vi "PPL_TRAJECTORY_EXECUTE_ABS.vi"(8 "Init":bool, 10 "Max Wheel Speed M/S":dbl, 11 "End Pose ENG":T6={"TRANSLATION"={"X"=0.0, "Y"=0.0}, "ROTATION"={"VALUE"=0.0, "COS"=1.0, "SIN"=0.0}} {"ROTATION"."SIN" format="%13.4f"; "ROTATION"."COS" format="%13.4f"; "ROTATION"."VALUE" format="%13.4f"; "TRANSLATION"."Y" format="%14.3f"; "TRANSLATION"."X" format="%14.3f"}) -> (0 "AtReference":bool, 2 "Right Speed Dmd M/S":dbl, 3 "Left Speed Dmd M/S":dbl)   [LabVIEW 2019]
uses:
  <vilib>/Rock Robotics/WPI/ThirdParty/JAS_Junk/TrajLib/TypeDef/POSE2D.ctl
  <vilib>/Rock Robotics/WPI/ThirdParty/JAS_Junk/TrajLib/TypeDef/TRANSLATION2D.ctl
  <vilib>/Rock Robotics/WPI/ThirdParty/JAS_Junk/TrajLib/TypeDef/ROTATION2D.ctl
  <vilib>/Rock Robotics/WPI/ThirdParty/MJansen/PathPlanner/TypeDef/PathPlannerTrajectory.ctl
  <vilib>/Rock Robotics/WPI/ThirdParty/MJansen/PathPlanner/TypeDef/PathPlannerTrajectoryState.ctl
  <vilib>/Rock Robotics/WPI/ThirdParty/MJansen/PathPlanner/TypeDef/PathPlannerPathConstraints.ctl
  <vilib>/Rock Robotics/WPI/ThirdParty/JAS_Junk/TrajLib/VI/Util_GetTime_U32.vi
  <vilib>/Rock Robotics/WPI/ThirdParty/JAS_Junk/TrajLib/Conv_Deg_Radians.vi
  <vilib>/Rock Robotics/WPI/ThirdParty/JAS_Junk/TrajLib/Rotation2d_GetRadians.vi
  <vilib>/Rock Robotics/WPI/ThirdParty/JAS_Junk/TrajLib/VI/Util_GetTime_U64.vi
  PPL_TRAJECTORY_GLOBALS.vi
  Diff_Drive_System/PPL_DRIVE_GLOBALS.vi
  <vilib>/Rock Robotics/WPI/ThirdParty/JAS_Junk/TrajLib/Trajectory_Library.lvlib
  <vilib>/Rock Robotics/WPI/ThirdParty/MJansen/PathPlanner/PathPlanner24.lvlib
panel:
  out "PathPlannerTrajectory":T1 {"States"."TargetHolonomicRotation"."SIN" format="%13.4f"; "States"."TargetHolonomicRotation"."COS" format="%13.4f"; "States"."TargetHolonomicRotation"."VALUE" format="%13.4f"; "States"."Heading"."SIN" format="%13.4f"; "States"."Heading"."COS" format="%13.4f"; "States"."Heading"."VALUE" format="%13.4f"; "States"."PositionMeters"."Y" format="%14.3f"; "States"."PositionMeters"."X" format="%14.3f"}
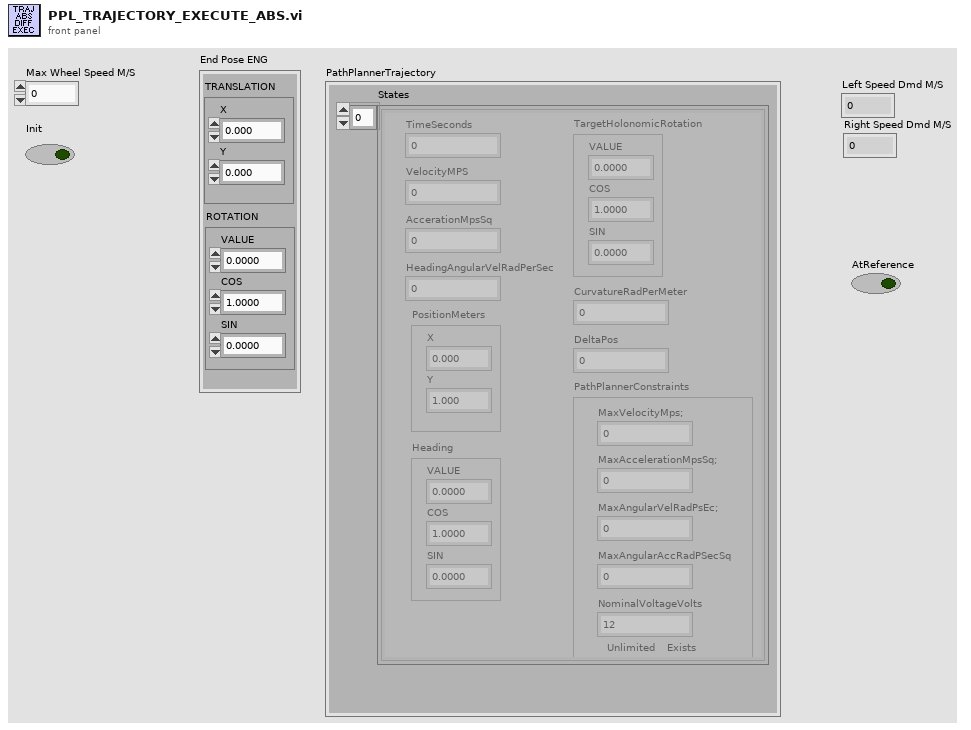
[diagram p1: front panel]
types:
  T1 = typedef "PathPlanner24.lvlib/PathPlannerTrajectory.ctl" = cluster{"States":T2[]}
  T2 = typedef "PathPlanner24.lvlib/PathPlannerTrajectoryState.ctl" = cluster{"TimeSeconds":dbl, "VelocityMPS":dbl, "AccerationMpsSq":dbl, "HeadingAngularVelRadPerSec":dbl, "PositionMeters":T3, "Heading":T4, "TargetHolonomicRotation":T4, "CurvatureRadPerMeter":dbl, "PathPlannerConstraints":T5, "DeltaPos":dbl}
  T3 = typedef "Trajectory_Library.lvlib/TRANSLATION2D.ctl" = cluster{"X":dbl, "Y":dbl}
  T4 = typedef "Trajectory_Library.lvlib/ROTATION2D.ctl" = cluster{"VALUE":dbl, "COS":dbl, "SIN":dbl}
  T5 = typedef "PathPlanner24.lvlib/PathPlannerPathConstraints.ctl" = cluster{"MaxVelocityMps;":dbl, "MaxAccelerationMpsSq;":dbl, "MaxAngularVelRadPsEc;":dbl, "MaxAngularAccRadPSecSq":dbl, "Exists":bool, "Unlimited":bool, "NominalVoltageVolts":dbl}
  T6 = typedef "Trajectory_Library.lvlib/POSE2D.ctl" = cluster{"TRANSLATION":T3, "ROTATION":T4}
  T7 = typedef "Trajectory_Library.lvlib/DIFF_DRIVE_KINEMATICS.ctl" = cluster{"TrackWidth_Meters":dbl}
  T8 = typedef "Trajectory_Library.lvlib/LTV_UNICYCLE_CONTROLLER_MODEL_PARAMS.CTL" = cluster{"Max linear ctrl effort M/S":dbl, "Max angular ctrl effort Rad/S":dbl, "Max Heading Meas Tol Rad":dbl, "Max X Pos Meas Tol M":dbl, "Max Y Pos Meas Tol M":dbl, "Max Linear Vel M/S":dbl}
  T9 = typedef "PathPlanner24.lvlib/PathPlannerCtrlLTVUnicycleConfig.ctl" = cluster{"Max Wheel Speed M/S":dbl, "Track Width M":dbl, "LTV_Unicycle_Ctrl_Model":T8, "LTV_Unicycle_Ctrl_Tolerance":T10}
  T10 = typedef "Trajectory_Library.lvlib/LTV_UNICYCLE_CONTROLLER_TOLERANCE.CTL" = cluster{"Max Heading Tolerance Rad":dbl, "Max X Tolerance M":dbl, "Max Y Tolerance M":dbl}
  T11 = typedef "Trajectory_Library.lvlib/LTV_UNICYCLE_CONTROLLER.ctl" = cluster{"States":i32, "Inputs":i32, "PoseError":T6, "PoseTolerance":T6, "Dt":dbl, "Enabled":bool, "LQR_K_Table":T12}
  T12 = typedef "Trajectory_Library.lvlib/FUNCTION_GENERATOR_MATRIX.ctl" = cluster{"Table Xs":dbl[], "Table Ys":variant[], "MinX":dbl, "MaxX":dbl, "ItemCount":i32, "Rows":i32, "Columns":i32}
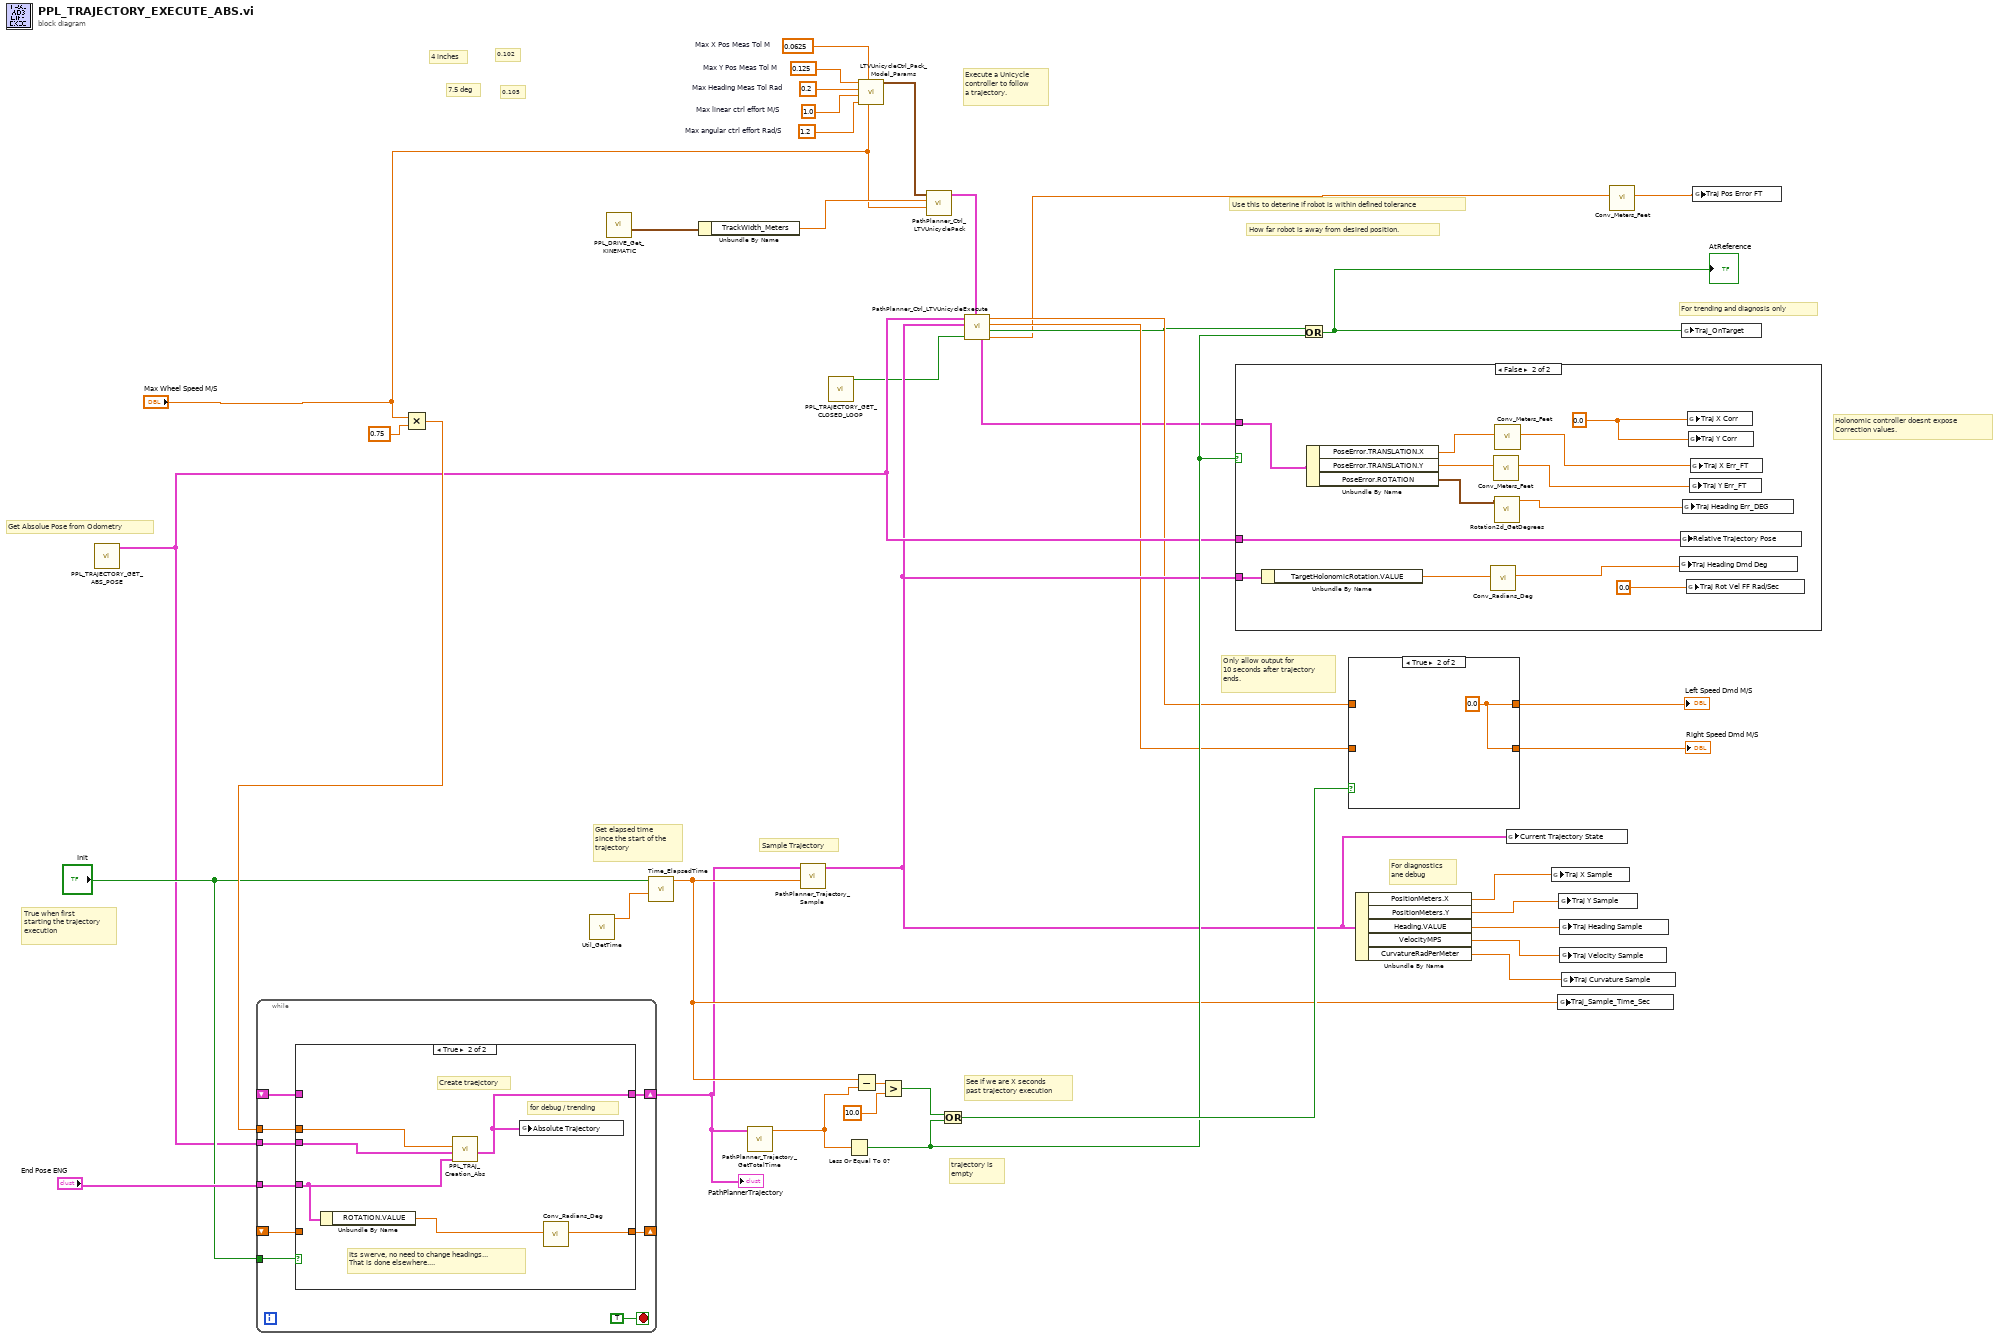
[diagram p0: block diagram]
diagram:
  w15 = 0.125  # Max Y Pos Meas Tol M
  w14 = 0.2  # Max Heading Meas Tol Rad
  w13 = 1.0  # Max linear ctrl effort M/S
  w12 = 1.2  # Max angular ctrl effort Rad/S
  w11 = 0.0625  # Max X Pos Meas Tol M
  # "0.105"
  # "0.102"
  # "Execute a Unicycle\ncontroller to follow\na trajectory."
  # "How far robot is away from desired position."
  # "Use this to deterine if robot is within defined tolerance"
  # "4 inches"
  # "7.5 deg"
  # "trajectory is \nempty"
  # "True when first\nstarting the trajectory\nexecution"
  # "Get elapsed time\nsince the start of the\ntrajectory"
  # "Holonomic controller doesnt expose\nCorrection values."
  # "For trending and diagnosis only"
  # "For diagnostics\nane debug"
  # "Get Absolue Pose from Odometry"
  # "Sample Trajectory"
  # "See if we are X seconds \npast trajectory execution"
  # "Only allow output for\n10 seconds after trajectory\nends."
  n1 = call "PPL_TRAJECTORY_GET_ABS_POSE.vi"() -> ("Absolute Odometry Pose"=w10:T6)  [unwired: 11 in]
  n2 = Multiply(x="Max Wheel Speed M/S", y=0.75) -> (x*y=w24:dbl)
  n3 = while {
    tunnel: "Init" -> [w48]
    tunnel: w10 -> [w47]
    shift-right: [w46] -> w26
    shift-left: _ -> [w45]
    shift-right: [w44] -> _
    shift-left: _ -> [w43]
    tunnel: "End Pose ENG" -> [w42]
    tunnel: w24 -> [w41]
    stop <- TRUE stop-if-true
    n4 = case shown="True" w48 {
      tunnel: w47 -> [_ w53]
      tunnel: [w51 w54] -> w46
      tunnel: w45 -> [w51 _]
      tunnel: [w50 w56] -> w44
      tunnel: w43 -> [w50 _]
      tunnel: w42 -> [_ w57]
      tunnel: w41 -> [_ w52]
      frame False {
      }
      frame True {
        # "for debug / trending"
        # "Its swerve, no need to change headings...\nThat is done elsewhere...."
        # "Create traejctory"
        n5 = Unbundle By Name(w57) -> ("ROTATION.VALUE"=w55:dbl)
        n6 = call "PPL_TRAJ_Creation_Abs.vi"("End Pose  ENG"=w57, "Current Pose SI"=w53, "Max Velocity M/S"=w52) -> ("PathPlannerTrajectory"=w54:T1)  [unwired: 6 in, 2 out]
        n7 = global write "PPL_TRAJECTORY_GLOBALS.vi" "Absolute Trajectory"(w54) -> ()
        n8 = call <vilib>:"Conv_Radians_Deg.vi"("Radians"=w55) -> ("Degrees"=w56:dbl)  [unwired: 10 in]
      }
    }
  }
  "PathPlannerTrajectory" <- w26
  n9 = call <vilib>:"Util_GetTime.vi"() -> ("FPGA_Time_Seconds"=w38:dbl)  [unwired: 9 in, 2 out]
  n10 = call "PPL_DRIVE_Get_KINEMATIC.vi"() -> ("out DIFF_DRIVE_KINEMATICS"=w21:T7)  [unwired: 11 in]
  n11 = call <vilib>:"Time_ElapsedTime.vi"("PassthroughTime_SEC"=w38, "Reset"="Init") -> ("Elapsed Time Sec"=w27:dbl)  [unwired: 9 in]
  n12 = Unbundle By Name(w21) -> ("TrackWidth_Meters"=w8:dbl)
  n13 = call <vilib>:"PathPlanner_Trajectory_GetTotalTime.vi"("PathPlannerTrajectory"=w26) -> ("TotalTimeSeconds"=w25:dbl)  [unwired: 10 in]
  n14 = call <vilib>:"PathPlanner_Trajectory_Sample.vi"("Time"=w27, "PathPlannerTrajectory"=w26) -> ("PathPlannerState"=w9:T2)  [unwired: 9 in]
  n15 = call "PPL_TRAJECTORY_GET_CLOSED_LOOP.vi"() -> ("AUTO_CLOSED_LOOP"=w7:bool)  [unwired: 11 in]
  n16 = Less Or Equal To 0?(x=w25) -> (x <= 0?=w28:bool)
  n17 = Subtract(x=w27, y=w25) -> (x-y=w40:dbl)
  n18 = call <vilib>:"LTVUnicycleCtrl_Pack_Model_Params.vi"("Max Linear Vel M/S"="Max Wheel Speed M/S", "Max X Pos Meas Tol M"=w11, "Max angular ctrl effort Rad/S"=w12, "Max linear ctrl effort M/S"=w13, "Max Heading Meas Tol Rad"=w14, "Max Y Pos Meas Tol M"=w15) -> ("LTV_Unicycle_Ctrl_Model _Params"=w17:T8)  [unwired: 5 in]
  n19 = Greater?(x=w40, y=10.0) -> (0:w31:bool)
  n20 = call <vilib>:"PathPlanner_Ctrl_LTVUnicyclePack.vi"("Max Speed M/S"="Max Wheel Speed M/S", "Track Width Meters"=w8, "LTV_Unicycle_Ctrl_Model"=w17) -> ("PathPlanner_Ctrl_LTVUnicycleConfig"=w16:T9)  [unwired: 8 in]
  n21 = Or(x=w31, y=w28) -> (x .or. y?=w30:bool)
  n22 = call <vilib>:"PathPlanner_Ctrl_LTVUnicycleExecute.vi"("PathPlanner_Ctrl_LTVUnicycle_Config"=w16, "Enabled"=w7, "PathPlannerState"=w9, "Current Pose SI"=w10) -> ("Position Error M"=w2:dbl, "At Reference"=w3:bool, "Normalized Right Wheel Dmd M/S"=w4:dbl, "Normalized Left Wheel Dmd M/S"=w5:dbl, "out LTV_UNICYCLE_CONTROLLER"=w1:T11)  [unwired: 3 in]
  n23 = case shown="False" w28 {
    tunnel: w10 -> [_ w61]
    tunnel: w9 -> [_ w64]
    tunnel: w1 -> [_ w58]
    frame True {
    }
    frame False {
      w70 = 0.0 ("Y Corr")
      n24 = Unbundle By Name(w64) -> ("TargetHolonomicRotation.VALUE"=w63:dbl)
      n25 = Unbundle By Name(w58) -> ("PoseError.TRANSLATION.X"=w66:dbl, "PoseError.TRANSLATION.Y"=w65:dbl, "PoseError.ROTATION"=w59:T4)
      n26 = call <vilib>:"Conv_Radians_Deg.vi"("Radians"=w63) -> ("Degrees"=w62:dbl)  [unwired: 10 in]
      n27 = call <vilib>:"Conv_Meters_Feet.vi"("Meters"=w65) -> ("Feet"=w69:dbl)  [unwired: 10 in]
      n28 = call <vilib>:"Rotation2d_GetDegrees.vi"("in ROTATION"=w59) -> ("AngleDegrees"=w60:dbl)  [unwired: 10 in]
      n29 = call <vilib>:"Conv_Meters_Feet.vi"("Meters"=w66) -> ("Feet"=w68:dbl)  [unwired: 10 in]
      n30 = global write "PPL_TRAJECTORY_GLOBALS.vi" "Traj Heading Dmd Deg"(w62) -> ()
      n31 = global write "PPL_TRAJECTORY_GLOBALS.vi" "Relative Trajectory Pose"(w61) -> ()
      n32 = global write "PPL_TRAJECTORY_GLOBALS.vi" "Traj Heading Err_DEG"(w60) -> ()
      n33 = global write "PPL_TRAJECTORY_GLOBALS.vi" "Traj Rot Vel FF Rad/Sec"(0.0 ("Traj Heading Dmd Deg")) -> ()
      n34 = global write "PPL_TRAJECTORY_GLOBALS.vi" "Traj X Corr"(w70) -> ()
      n35 = global write "PPL_TRAJECTORY_GLOBALS.vi" "Traj Y Corr"(w70) -> ()
      n36 = global write "PPL_TRAJECTORY_GLOBALS.vi" "Traj Y Err_FT"(w69) -> ()
      n37 = global write "PPL_TRAJECTORY_GLOBALS.vi" "Traj X Err_FT"(w68) -> ()
    }
  }
  n38 = Or(x=w3, y=w28) -> (x .or. y?=w29:bool)
  "AtReference" <- w29
  n39 = case shown="True" w30 {
    tunnel: w5 -> [w72 _]
    tunnel: [w72 w73] -> w20
    tunnel: w4 -> [w71 _]
    tunnel: [w71 w73] -> w19
    frame False {
    }
    frame True {
      w73 = 0.0 ("vX")
    }
  }
  "Left Speed Dmd M/S" <- w20
  "Right Speed Dmd M/S" <- w19
  n40 = Unbundle By Name(w9) -> ("PositionMeters.X"=w37:dbl, "PositionMeters.Y"=w36:dbl, "Heading.VALUE"=w35:dbl, "VelocityMPS"=w34:dbl, "CurvatureRadPerMeter"=w33:dbl)
  n41 = global write "PPL_TRAJECTORY_GLOBALS.vi" "Current Trajectory State"(w9) -> ()
  n42 = global write "PPL_TRAJECTORY_GLOBALS.vi" "Traj X Sample"(w37) -> ()
  n43 = global write "PPL_TRAJECTORY_GLOBALS.vi" "Traj_Sample_Time_Sec"(w27) -> ()
  n44 = global write "PPL_TRAJECTORY_GLOBALS.vi" "Traj Y Sample"(w36) -> ()
  n45 = global write "PPL_TRAJECTORY_GLOBALS.vi" "Traj Heading Sample"(w35) -> ()
  n46 = global write "PPL_TRAJECTORY_GLOBALS.vi" "Traj Velocity Sample"(w34) -> ()
  n47 = global write "PPL_TRAJECTORY_GLOBALS.vi" "Traj Curvature Sample"(w33) -> ()
  n48 = call <vilib>:"Conv_Meters_Feet.vi"("Meters"=w2) -> ("Feet"=w18:dbl)  [unwired: 10 in]
  n49 = global write "PPL_TRAJECTORY_GLOBALS.vi" "Traj_OnTarget"(w29) -> ()
  n50 = global write "PPL_TRAJECTORY_GLOBALS.vi" "Traj Pos Error FT"(w18) -> ()
